vi "dotest.vi"() -> ()   [LabVIEW 2015]
panel:
  out "error out":errorcluster
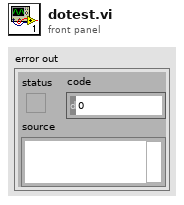
[diagram p1: front panel]
types:
  T1 = enum16{"init", "config", "start", "write", "stop"}
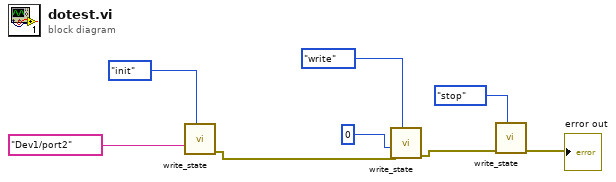
[diagram p0: block diagram]
diagram:
  n1 = call "write_state.vi"("Enum"=T1."init", "lines"=tag "Dev1/port2") -> ("error out"=w1:errorcluster)  [unwired: 8 in]
  n2 = call "write_state.vi"("Enum"=T1."write", "error in"=w1, "data"=u8 0) -> ("error out"=w4:errorcluster)  [unwired: 7 in]
  n3 = call "write_state.vi"("Enum"=T1."stop", "error in"=w4) -> ("error out"=→"error out":errorcluster)  [unwired: 8 in]
